vi "Update Gyro.vi"(11 "Gyro ID (1 or 2)":i32) -> ()   [LabVIEW 2015]
doc: "Updates the gyro bias/angle. This is a required block and should be placed in Periodic Tasks."
uses:
  Gyro Global.vi
panel:
  out "x-y":u32
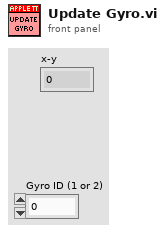
[diagram p1: front panel]
types:
  T1 = typedef "WPI_AnalogChannelDevRef.ctl" = cluster{"DevStatus":errorcluster, "Analog Channel":T2}
  T2 = typedef "FPGA_AIChannel.ctl" = enum8{"AI 0", "AI 1", "AI 2", "AI 3", "AI MXP 0", "AI MXP 1", "AI MXP 2", "AI MXP 3", "Invalid"}
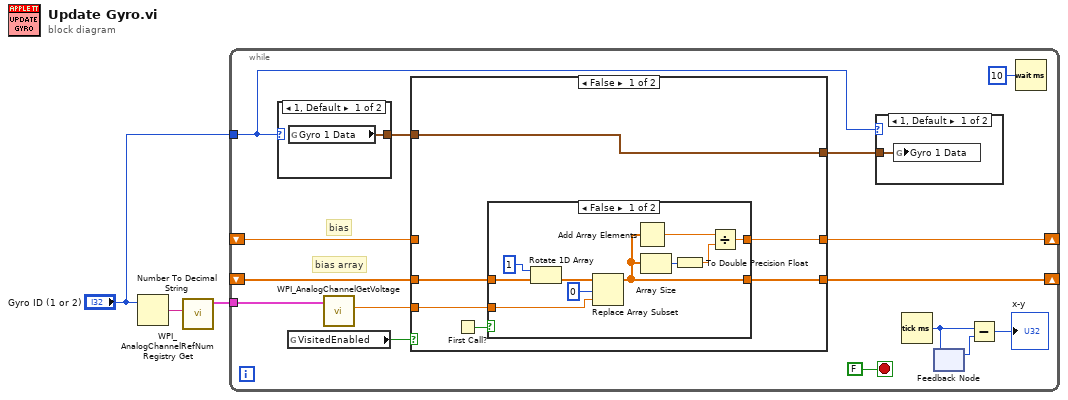
[diagram p0: block diagram]
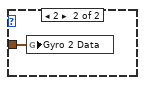
[diagram p2: hidden frame]
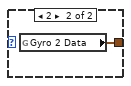
[diagram p3: hidden frame]
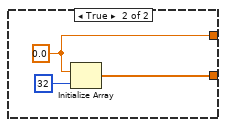
[diagram p4: hidden frame]
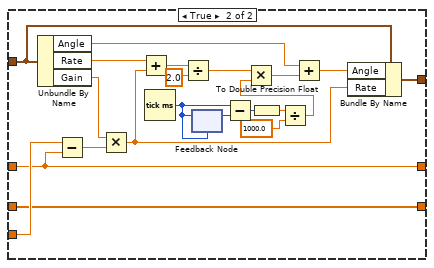
[diagram p5: hidden frame]
diagram:
  n1 = Number To Decimal String(number="Gyro ID (1 or 2)") -> (decimal integer string=w2:string)  [unwired: 1 in]
  n2 = call <vilib>:"WPI_AnalogChannelRefNum Registry Get.vi"("refnum name"=w2) -> ("AIDeviceRef"=w3:T1)  [unwired: 9 in, 1 out]
  n3 = while {
    shift-right: [w16] -> _
    shift-left: _ -> [w15]
    shift-right: [w10] -> _
    shift-left: _ -> [w13]
    tunnel: w3 -> [w12]
    tunnel: "Gyro ID (1 or 2)" -> [w7]
    stop <- FALSE stop-if-true
    # "bias"
    # "bias array"
    n4 = case shown="1, Default" w7 {
      tunnel: [w21 w22] -> w9
      frame 1, Default {
        n5 = global read "Gyro Global.vi" "Gyro 1 Data"() -> (w21:cluster{"Rate":dbl, "Angle":dbl, "Gain":dbl})
      }
      frame 2 {
        n6 = global read "Gyro Global.vi" "Gyro 2 Data"() -> (w22:cluster{"Rate":dbl, "Angle":dbl, "Gain":dbl})
      }
    }
    n7 = global read "Gyro Global.vi" "VisitedEnabled"() -> (w14:bool)
    n8 = call <vilib>:"WPI_AnalogChannelGetVoltage.vi"("AIDeviceRef"=w12) -> ("Voltage"=w11:dbl)  [unwired: 8 in, 2 out]
    n9 = case shown="False" w14 {
      tunnel: [w27 w61] -> w16
      tunnel: w15 -> [w26 w61]
      tunnel: [w25 w60] -> w10
      tunnel: w9 -> [w23 w57]
      tunnel: w11 -> [w24 w62]
      tunnel: w13 -> [_ w60]
      tunnel: [w23 w56] -> w8
      frame False {
        n10 = First Call?() -> (First Call?: T/F=w28:bool)
        n11 = case shown="False" w28 {
          tunnel: [w31 w40] -> w27
          tunnel: w26 -> [w38 _]
          tunnel: [w33 w39] -> w25
          tunnel: w24 -> [w30 _]
          frame False {
            n12 = Rotate 1D Array(1:w38, 2:1 ("n")) -> (0:w32:dbl[])
            n13 = Replace Array Subset(array=w32, new element=w30, index=0) -> (w31:dbl[])
            n14 = Add Array Elements(numeric array=w31) -> (sum=w36:dbl)
            n15 = Array Size(array=w31) -> (size(s)=w35:i32)
            n16 = To Double Precision Float(number=w35) -> (double precision float=w34:dbl)
            n17 = Divide(x=w36, y=w34) -> (x/y=w33:dbl)
          }
          frame True {
            w39 = 0.0 ("element")
            n18 = Initialize Array(w39, 32 ("dimension size")) -> (w40:dbl[])
          }
        }
      }
      frame True {
        n19 = Unbundle By Name(w57) -> ("Angle"=w43:dbl, "Rate"=w54:dbl, "Gain"=w58:dbl)
        n20 = Subtract(x=w62, y=w60) -> (x-y=w59:dbl)
        n21 = Multiply(x=w58, y=w59) -> (x*y=w55:dbl)
        n22 = Add(x=w54, y=w55) -> (x+y=w53:dbl)
        n23 = Tick Count (ms)() -> (millisecond timer value=w50:u32)
        n24 = Divide(x=w53, y=2.0) -> (x/y=w51:dbl)
        n25 = feedback-in #1(w50) -> ()
        n26 = feedback #1(w50) -> (w49:u32)
        n27 = Subtract(x=w50, y=w49) -> (x-y=w48:u32)
        n28 = To Double Precision Float(number=w48) -> (double precision float=w47:dbl)
        n29 = Divide(x=w47, y=1000.0) -> (x/y=w45:dbl)
        n30 = Multiply(x=w51, y=w45) -> (x*y=w44:dbl)
        n31 = Add(x=w43, y=w44) -> (x+y=w42:dbl)
        n32 = Bundle By Name(cluster=w57, "Angle"=w42, "Rate"=w55) -> (w56:cluster{"Rate":dbl, "Angle":dbl, "Gain":dbl})
      }
    }
    n33 = case shown="1, Default" w7 {
      tunnel: w8 -> [w19 w20]
      frame 1, Default {
        n34 = global write "Gyro Global.vi" "Gyro 1 Data"(w19) -> ()
      }
      frame 2 {
        n35 = global write "Gyro Global.vi" "Gyro 2 Data"(w20) -> ()
      }
    }
    n36 = Tick Count (ms)() -> (millisecond timer value=w6:u32)
    n37 = feedback-in #2(w6) -> ()
    n38 = feedback #2() -> (w5:u32)  [unwired: 1 in]
    n39 = Subtract(x=w6, y=w5) -> (x-y=→"x-y":u32)
    n40 = Wait (ms)(milliseconds to wait=u32 10) -> ()  [unwired: 1 out]
  }
